vi "Stop.vi"(8 "error in":errorcluster, 11 "DAQmx Base CFG in":refnum<class "DAQmx Base CFG.lvclass">) -> (0 "error out":errorcluster, 3 "DAQmx Base CFG out":refnum<class "DAQmx Base CFG.lvclass">)   [LabVIEW 2023, in "DAQmx Base CFG.lvclass"]
uses:
  DAQmx Base CFG.lvclass
  Configurations/CFG Base/CFG Base.lvclass/CFG Base.ctl
  DAQmx Base CFG.lvclass/DAQmx Base CFG.ctl
  Configurations/CFG Base/CFG Base.lvclass
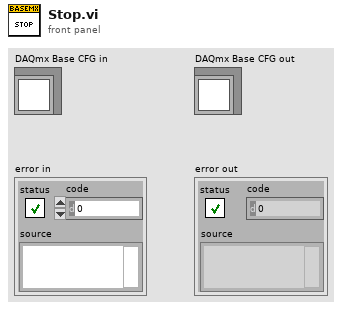
[diagram p1: front panel]
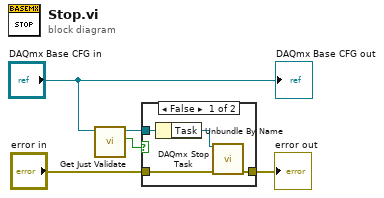
[diagram p0: block diagram]
diagram:
  n1 = call "Get Just Validate.vi"("CFG Base in"="DAQmx Base CFG in") -> ("Just Validate"=w1:bool, "CFG Base out"=w3:refnum<class "DAQmx Base CFG.lvclass">)  [unwired: 9 in]
  n2 = case shown="False" w1 {
    tunnel: w3 -> [w8 _]
    tunnel: [w7 w10] -> w5
    tunnel: "error in" -> [w6 w10]
    frame False {
      n3 = Unbundle By Name(w8) -> ("Task"=w9:refnum<k21>)
      n4 = call <vilib>:"DAQmx Stop Task.vi"("task/channels in"=w9, "error in"=w6) -> ("error out"=w7:errorcluster)  [unwired: 12 in, 1 out]
    }
    frame True {
    }
  }
  "error out" <- w5
  "DAQmx Base CFG out" <- "DAQmx Base CFG in"
